vi "AWG Write Waveforms.vi"(0 "Semiconductor Module Context":T1, 1 "VHi":dbl=50.0, 2 "Vlo":dbl, 3 "AmpGain":dbl=15.0 format="%#_13g", 4 "Amplitude":dbl, 5 "error in (no error)":errorcluster, 7 "Pins":string[](array[string]), 9 "Waveform Name":string="myWaveform") -> (6 "Gain":dbl, 8 "Offset":dbl, 10 "Waveform Amplitude":dbl, 14 "Semiconductor Module Context Out":T1, 19 "error out":errorcluster)   [LabVIEW 2013]
uses:
  <vilib>/NI_TestStand_SemiconductorModule/NI_TestStand_Semiconductor_Module.lvlibp/PinMap/General/SemiconductorModuleContext.ctl
  <instrlib>/niFgen/niFgen.llb/niFgen Output Mode.ctl
  <instrlib>/niFgen/niFgen.llb/niFgen Write Named Waveform (I16).vi
  <vilib>/NI_TestStand_SemiconductorModule/NI_TestStand_Semiconductor_Module.lvlibp
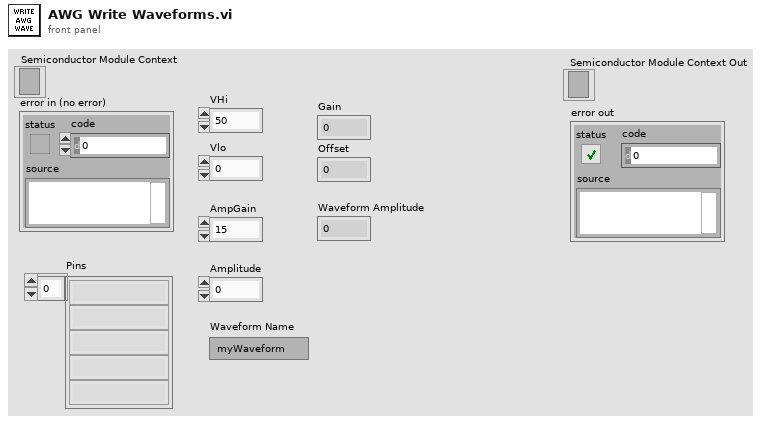
[diagram p1: front panel]
types:
  T1 = typedef "NI_TestStand_Semiconductor_Module.lvlibp/SemiconductorModuleContext.ctl" = refnum<k7>
  T2 = cluster{"Waveform Type":u16, "Amplitude":dbl, "# of Points":u32}
  T3 = typedef "niFgen Output Mode.ctl" = u32
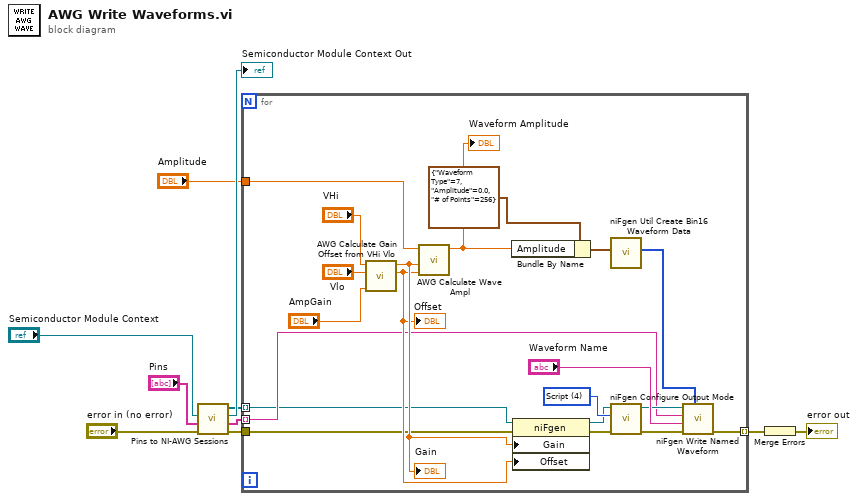
[diagram p0: block diagram]
diagram:
  n1 = call "Pins to NI-AWG Sessions.vi"("error in (no error)"="error in (no error)", "Pins"="Pins", "Semiconductor Module Context"="Semiconductor Module Context") -> ("error out"=w4:errorcluster, "Channel Lists"=w6:string[], "Semiconductor Module Context Out"=→"Semiconductor Module Context Out":T1, "Instrument Sessions"=w5:refnum<k15>[])  [unwired: 5 in]
  n2 = for {
    tunnel: w6 -> [w14] mode=indexing
    tunnel: w5 -> [w13] mode=indexing
    tunnel: w4 -> [w12]
    tunnel: "Amplitude" -> [w27]
    tunnel: [w11] -> w1 mode=indexing
    w26 = T3 4 items=["Standard Function", "Frequency List", "Arbitrary Waveform", "Arbitrary Sequence", "Script"] ("Output Mode (default: 0=Standard Function)")
    n3 = call "AWG Calculate Gain Offset from VHi Vlo.vi"("AmpGain"="AmpGain", "Vlo"="Vlo", "VHi"="VHi") -> ("Offset"=w16:dbl, "Gain"=w17:dbl)  [unwired: 6 in, 1 out]
    "Gain" <- w17
    "Offset" <- w16
    n4 = call "AWG Calculate Wave Ampl.vi"("Offset"=w16, "Gain"=w17, "Amplitude"=w27) -> ("Waveform Amplitude"=w15:dbl)  [unwired: 8 in]
    "Waveform Amplitude" <- w15
    n5 = Bundle By Name(cluster=T2 {"Waveform Type"=7, "Amplitude"=0.0, "# of Points"=256} ("Waveform"), "Amplitude"=w15) -> (w18:T2)
    n6 = property class="niFgen"(reference=w13, error in=w12, "Gain"=w17, "Offset"=w16) -> (reference out=w21:refnum<k15>, error out=w20:errorcluster)
    n7 = call <instrlib>:"niFgen Util Create Bin16 Waveform Data.vi"("Waveform"=w18) -> ("Waveform Data"=w25:i16[])  [unwired: 10 in]
    n8 = call <instrlib>:"niFgen Configure Output Mode.vi"("error in (no error)"=w20, "Output Mode (default: 0=Standard Function)"=w26, "Instrument Handle"=w21) -> ("error out"=w23:errorcluster, "Instrument Handle Out"=w22:refnum<k15>)  [unwired: 6 in]
    n9 = call-poly <instrlib>:"niFgen Write Named Waveform.vi"("Waveform Data"=w25, "error in (no error)"=w23, "Waveform Name"="Waveform Name", "Channel Name"=w14, "Instrument Handle"=w22) -> ("error out"=w11:errorcluster)  [unwired: 4 in, 2 out]
  }
  n10 = Merge Errors(w1) -> (→"error out":errorcluster)
